vi "MGI Decimate Array with Offset (DBL[]).vi"(8 "error in (no error)":errorcluster, 9 "Offset":i32, 10 "Decimation":i32, 11 "Double[] In":dbl[](array[numeric])) -> (0 "error out":errorcluster, 3 "Double[] Out":dbl[](array[numeric]))   [LabVIEW 2016]
doc: "Decimates the specified array by the specified amount. \"Offset\" specifies which decimation is output. This occurs even if the following error occur:\nAn error is output if the array length is not an integer multiple of the decimation. \nAn error is output if Offset is greater than or equal to the Decimation.\n\nAuthored by Shawn Walpole\nsupport@mooregoodideas.com\nwww.mooregoodideas.com\n\nCopyright (c) 2010, Moore Good Ideas, Inc.\n\nAll rights reserved.\n\nRedistribution and use in source and binary forms, with or without modification, are permitted provided that the following conditions are met:\n\n * Redistributions of source code must retain the above copyright notice, this list of conditions and the following disclaimer.\n * Redistributions in binary form must reproduce the above copyright notice, this list of conditions and the following disclaimer in the documentation and/or other materials provided with the distribution.\n * Neither the name of Moore Good Ideas, Inc. nor the names of its contributors may be used to endorse or promote products derived from this software without specific prior written permission.\n\nTHIS SOFTWARE IS PROVIDED BY THE COPYRIGHT HOLDERS AND CONTRIBUTORS \"AS IS\" AND ANY EXPRESS OR IMPLIED WARRANTIES, INCLUDING, BUT NOT LIMITED TO, THE IMPLIED WARRANTIES OF MERCHANTABILITY AND FITNESS FOR A PARTICULAR PURPOSE ARE DISCLAIMED. IN NO EVENT SHALL THE COPYRIGHT OWNER OR CONTRIBUTORS BE LIABLE FOR ANY DIRECT, INDIRECT, INCIDENTAL, SPECIAL, EXEMPLARY, OR CONSEQUENTIAL DAMAGES (INCLUDING, BUT NOT LIMITED TO, PROCUREMENT OF SUBSTITUTE GOODS OR SERVICES; LOSS OF USE, DATA, OR PROFITS; OR BUSINESS INTERRUPTION) HOWEVER CAUSED AND ON ANY THEORY OF LIABILITY, WHETHER IN CONTRACT, STRICT LIABILITY, OR TORT (INCLUDING NEGLIGENCE OR OTHERWISE) ARISING IN ANY WAY OUT OF THE USE OF THIS SOFTWARE, EVEN IF ADVISED OF THE POSSIBILITY OF SUCH DAMAGE."
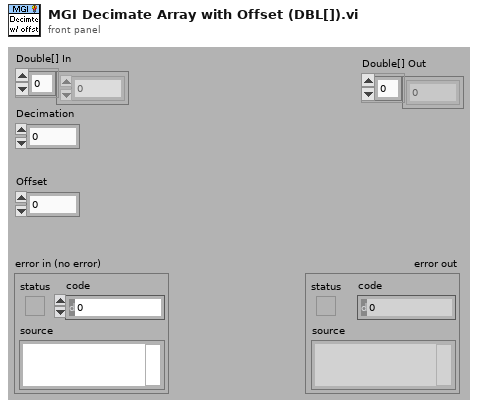
[diagram p1: front panel]
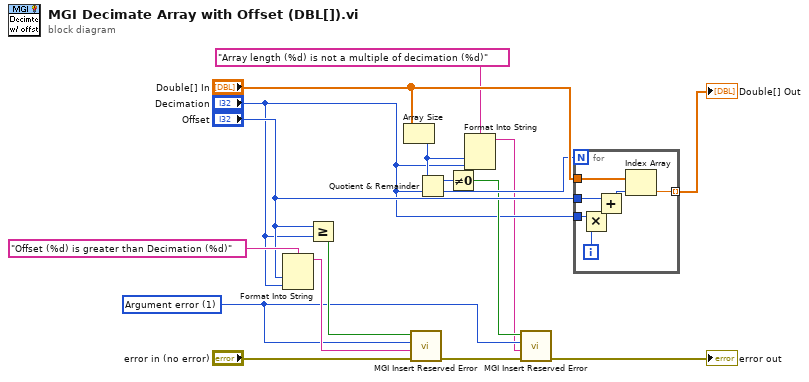
[diagram p0: block diagram]
diagram:
  w6 = u16 1 items=["No error", "Argument error", "Memory is full", "Out of zone", "End of file", "File already open", "Generic file I/O error", "File not found", "File permission error", "Disk is full", "Duplicate path", "Too many files open", "System feature not enabled", "Resource file not found", "Cannot add resource", "Resource not found", "Image not found", "Image memory error", "Pen does not exist", "Config type invalid", "Config token not found", "Config parse error", "Config memory error", "Bad external code format", "Bad external code offset", "External code not present", "Null window", "Destroy window error", "Null menu", "Print aborted", "Bad print record", "Print driver error", "Windows error during printing", "Memory error during printing", "Print dialog error", "Generic print error", "Invalid device refnum", "Device not found", "Device parameter error", "Device unit error", "Cannot open device", "Device call aborted", "Generic error", "Cancelled by user", "Object ID too low", "Object ID too high", "Object not in heap", "Unknown heap", "Unknown object (invalid DefProc)", "Unknown object (DefProc not in table)", "Message out of range", "Invalid (null) method", "Unknown message", "Manager call not supported", "Bad address", "Network operation in progress", "Network operation timed out", "Connection is busy", "Network attribute not supported", "Network error", "Address in use", "System out of memory", "Connection aborted", "Connection refused", "Not connected", "Already connected", "Connection closed", "Initialization error (interapplication manager)", "Bad occurrence", "Wait on unbound occurrence handler", "Occurrence queue overflow", "Datalog type conflict", "Unused", "Unrecognized type (interapplication manager)", "Memory corrupt", "Failed to make temporary DLL", "Old CIN version", "Drag socket not found", "Failed to load drop-object", "Failed to register OLE object", "Failed to release OLE object", "Format specifier type mismatch", "Unknown format specifier", "Too few format specifiers", "Too many format specifiers", "Scan failed", "Newer CIN version", "OLE Convert", "Runtime menu error", "Password tampered", "Unknown error code"] ("Reserved Error Code")
  n1 = Format Into String(format string="Offset (%d) is greater than Decimation (%d)", "Offset", "Decimation") -> (resulting string=w10:string)  [unwired: 2 in, 1 out]
  n2 = Greater Or Equal?(x="Offset", y="Decimation") -> (x >= y?=w13:bool)
  n3 = Array Size(array="Double[] In") -> (size(s)=w4:i32)
  n4 = call <userlib>:"MGI Insert Reserved Error.vi"("Error In"="error in (no error)", "Error Description"=w10, "Reserved Error Code (Generic error)"=w6, "Error? (T)"=w13) -> ("Error Out"=w8:errorcluster)  [unwired: 7 in]
  n5 = Quotient & Remainder(x=w4, y="Decimation") -> (x-y*floor(x/y)=w5:i32, floor(x/y)=w16:i32)
  n6 = Not Equal To 0?(x=w5) -> (x != 0?=w9:bool)
  n7 = Format Into String(format string="Array length (%d) is not a multiple of decimation (%d)", w4, "Decimation") -> (resulting string=w1:string)  [unwired: 2 in, 1 out]
  n8 = call <userlib>:"MGI Insert Reserved Error.vi"("Error In"=w8, "Error Description"=w1, "Reserved Error Code (Generic error)"=w6, "Error? (T)"=w9) -> ("Error Out"=→"error out":errorcluster)  [unwired: 7 in]
  n9 = for {
    N: w16 -> [_]
    tunnel: "Decimation" -> [w23]
    tunnel: "Offset" -> [w22]
    tunnel: "Double[] In" -> [w20]
    tunnel: [w18] -> w15 mode=indexing
    i -> [w24]
    n10 = Multiply(x=w23, y=w24) -> (x*y=w21:i32)
    n11 = Add(x=w22, y=w21) -> (x+y=w19:i32)
    n12 = Index Array(array=w20, index=w19) -> (element=w18:dbl)
  }
  "Double[] Out" <- w15
